vi "Open and Write CSV File.vi"(0 "File Path Control":path, 7 "Header":string[](array[string]), 11 "Error In":errorcluster) -> (4 "Refnum Out":refnum<file>, 15 "Error Out":errorcluster)   [LabVIEW 2019]
doc: "This VI opens or creates a file refum depending on the file path comntrol input. This reference is then output from the VI. It also will write a header to csv file. If file already exists, header will be appended to the end of file. A string array is used to create string values for the header."
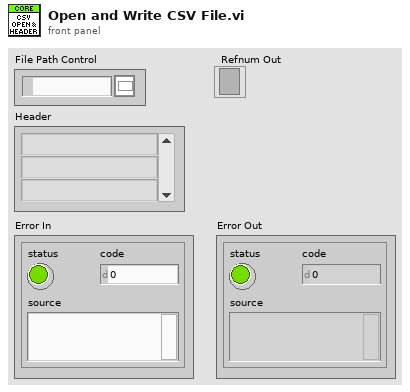
[diagram p1: front panel]
types:
  T1 = enum16{"open", "replace", "create", "open or create", "replace or create", "replace or create with confirmation"}
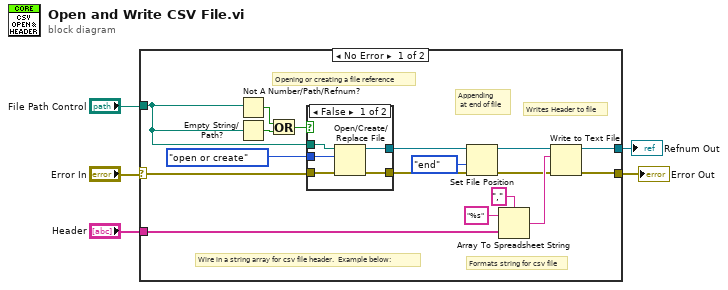
[diagram p0: block diagram]
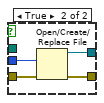
[diagram p2: hidden frame]
diagram:
  n1 = case shown="No Error" "Error In" {
    selector: "Error In" -> [w13 w32]
    tunnel: "File Path Control" -> [w14 _]
    tunnel: [w22 _] -> w1
    tunnel: [w12 w32] -> w3
    tunnel: "Header" -> [w6 _]
    frame No Error {
      # "Writes Header to file"
      # "Appending\n at end of file"
      # "Formats string for csv file"
      # "Opening or creating a file reference"
      # "Wire in a string array for csv file header.  Example below:"
      n2 = Not A Number/Path/Refnum?(number/path/refnum=w14) -> (NaN/Path/Refnum?=w18:bool)
      n3 = Empty String/Path?(string/path=w14) -> (empty?=w17:bool)
      n4 = Or(x=w18, y=w17) -> (x .or. y?=w16:bool)
      n5 = case shown="False" w16 {
        tunnel: T1."open or create" ("operation (0:open)") -> [w25 w31]
        tunnel: [w26 w30] -> w8
        tunnel: w14 -> [w27 _]
        tunnel: w13 -> [w24 w29]
        tunnel: [w23 w28] -> w11
        frame False {
          n6 = Open/Create/Replace File(file path (use dialog)=w27, error in=w24, operation (0:open)=w25) -> (refnum out=w26:refnum<file>, error out=w23:errorcluster)  [unwired: 3 in, 1 out]
        }
        frame True {
          n7 = Open/Create/Replace File(error in=w29, operation (0:open)=w31) -> (refnum out=w30:refnum<file>, error out=w28:errorcluster)  [unwired: 4 in, 1 out]
        }
      }
      n8 = Set File Position(refnum=w8, from (0:start)=enum16{"start", "end", "current"}."end", error in=w11) -> (refnum out=w7:refnum<file>, error out=w10:errorcluster)  [unwired: 1 in]
      n9 = Array To Spreadsheet String(delimiter (Tab)=",", array=w6, 3:"%s" ("format string")) -> (spreadsheet string=w19:string)
      n10 = Write to Text File(file (use dialog)=w7, text=w19, error in=w10) -> (refnum out=w22:refnum<file>, error out=w12:errorcluster)  [unwired: 1 in, 1 out]
    }
    frame Error {
    }
  }
  "Error Out" <- w3
  "Refnum Out" <- w1
